vi "Exercise 2.2 - Data.vi"() -> ()   [LabVIEW 2024]
panel:
  out "Unfiltered":dynamicdata(graph)
  out "Frequency":dbl
  out "Amplitude":dbl
  in  "stop":bool
  out "Filtered Signal":dynamicdata(graph)
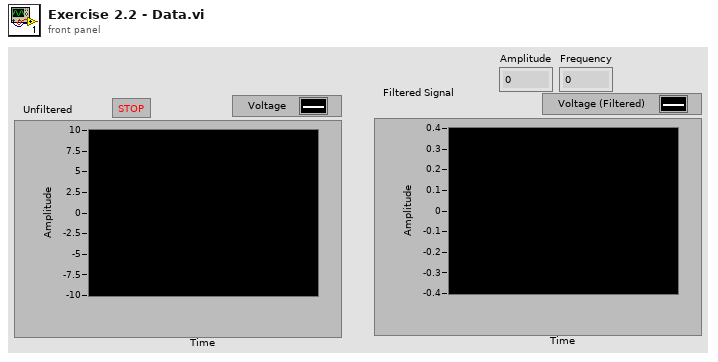
[diagram p1: front panel]
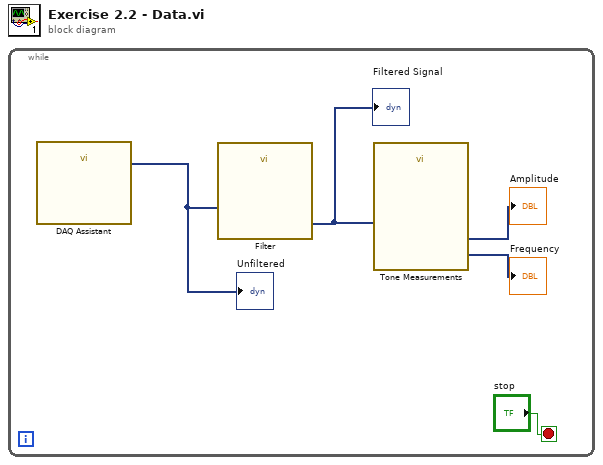
[diagram p0: block diagram]
diagram:
  n1 = while {
    stop <- "stop" stop-if-true
    n2 = call "DAQ Assistant"() -> ("data"=w1:dynamicdata)  [unwired: 16 in, 3 out]
    "Unfiltered" <- w1
    n3 = call "Filter"("Signal"=w1) -> ("Filtered Signal"=w2:dynamicdata)  [unwired: 9 in, 1 out]
    "Filtered Signal" <- w2
    n4 = call "Tone Measurements"("Signals"=w2) -> ("Frequency"=→"Frequency":dynamicdata, "Amplitude"=→"Amplitude":dynamicdata)  [unwired: 8 in, 1 out]
  }
